vi "Get Batch data.vi"(9 "Data":variant, 10 "Maps in":T2, 11 "Refnum in":T1) -> (1 "Maps out":T2, 2 "BatchData":string[](array[string]), 3 "Refnum out":T1)   [LabVIEW 2024]
uses:
  CTRLS/Maps.ctl
  CTRLS/BatchInfo.ctl
  CTRLS/Batch recipes.ctl
  <vilib>/addons/database/Connection.llb/Conn ObjectReference.ctl
  CTRLS/DB operation Selector.ctl
  <vilib>/addons/database/NI_Database_API.lvlib
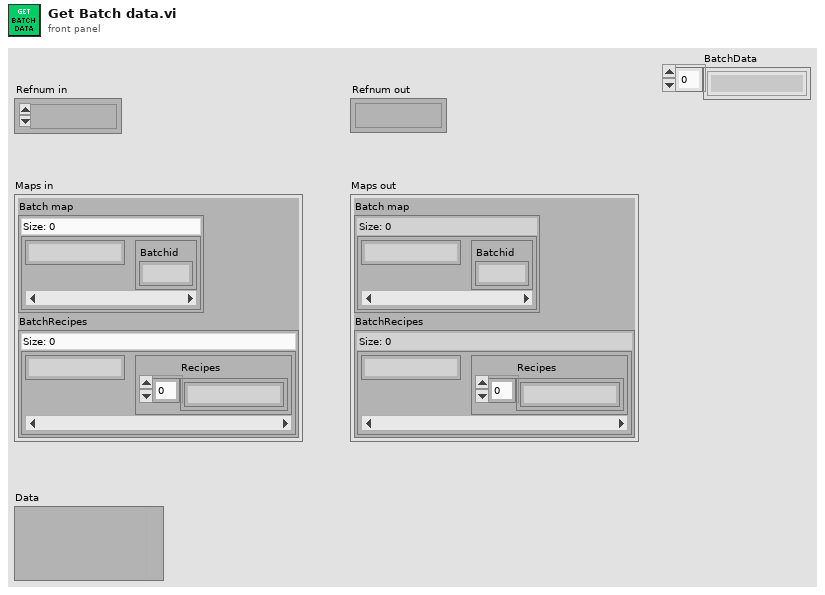
[diagram p1: front panel]
types:
  T1 = typedef "NI_Database_API.lvlib/Conn ObjectReference.ctl" = refnum<k1>
  T2 = typedef "Maps.ctl" = cluster{"Batch map":map{string, T3}, "BatchRecipes":map{string, T4}}
  T3 = typedef "BatchInfo.ctl" = cluster{"Batchid":i32}
  T4 = typedef "Batch recipes.ctl" = cluster{"Recipes":string[]}
  T5 = typedef "DB operation Selector.ctl" = enum16{"Select", "Insert", "Update", "Execute select Query", "Execute update query"}
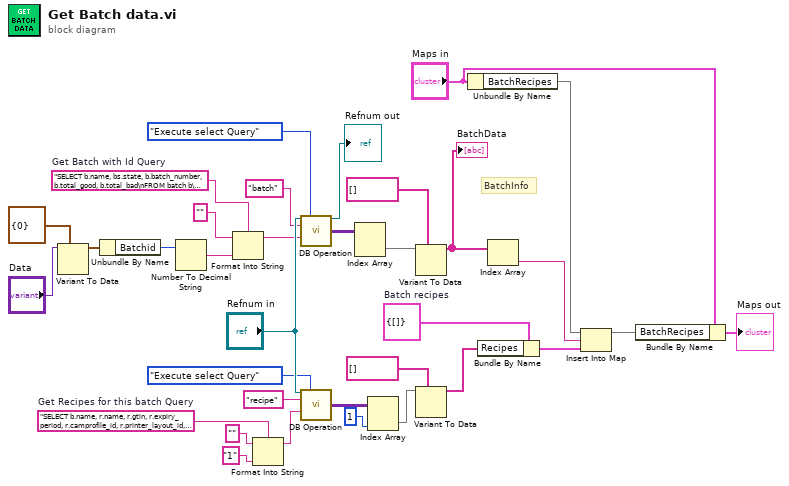
[diagram p0: block diagram]
diagram:
  w32 = T4 {"Recipes"=[]}  # Batch recipes
  w20 = "SELECT b.name, r.name, r.gtin, r.expiry_period, r.camprofile_id, r.printer_layout_id, r.roller_code\nFROM recipe r\nINNER JOIN batch b ON r.batch_id = b.id\nwhere r.batch_id = %s;"  # Get Recipes for this batch Query
  w7 = "SELECT b.name, bs.state, b.batch_number, b.total_good, b.total_bad\nFROM batch b\nINNER JOIN batch_state bs ON b.state_id = bs.id\nwhere b.id = %s;"  # Get Batch with Id Query
  # "BatchInfo"
  n1 = Variant To Data(type=T3 {"Batchid"=0} ("value"), Variant="Data") -> (data=w12:T3)  [unwired: 1 in, 1 out]
  n2 = Unbundle By Name(w12) -> ("Batchid"=w13:i32)
  n3 = Number To Decimal String(number=w13) -> (decimal integer string=w14:string)  [unwired: 1 in]
  n4 = Format Into String(format string=w7, initial string="", w14) -> (resulting string=w8:string)  [unwired: 1 in, 1 out]
  n5 = Format Into String(format string=w20, initial string="", "1" ("input 1")) -> (resulting string=w15:string)  [unwired: 1 in, 1 out]
  n6 = call "DB Operation.vi"("connection reference"="Refnum in", "DB Op Selector"=DB_operation_Selector."Execute select Query", "table"="batch", "SQL Query"=w8) -> ("connection reference out"=→"Refnum out":T1, "data out"=w5:variant[][])  [unwired: 9 in, 1 out]
  n7 = call "DB Operation.vi"("connection reference"="Refnum in", "DB Op Selector"=DB_operation_Selector."Execute select Query", "table"="recipe", "SQL Query"=w15) -> ("data out"=w16:variant[][])  [unwired: 9 in, 2 out]
  n8 = Index Array(array=w5) -> (element=w6:variant[])  [unwired: 2 in]
  n9 = Index Array(array=w16, index (col)=1 ("disabled index (col)")) -> (element=w17:variant[])  [unwired: 1 in]
  n10 = Variant To Data(type=string[] [], Variant=w6) -> (data=w9:string[])  [unwired: 1 in, 1 out]
  "BatchData" <- w9
  n11 = Variant To Data(type=string[] [], Variant=w17) -> (data=w34:string[])  [unwired: 1 in, 1 out]
  n12 = Unbundle By Name("Maps in") -> ("BatchRecipes"=w29:map{string, T4})
  n13 = Bundle By Name(cluster=w32, "Recipes"=w34) -> (w33:T4)
  n14 = Index Array(array=w9) -> (element=w31:string)  [unwired: 1 in]
  n15 = Insert Into Map(map in=w29, key=w31, value=w33) -> (map out=w30:map{string, T4})  [unwired: 2 out]
  n16 = Bundle By Name(cluster="Maps in", "BatchRecipes"=w30) -> (→"Maps out":T2)
